vi "Change Sensitivity.vi"(0 "Model in":refnum<class "Model.lvclass">, 5 "Channel":u8, 7 "Offset":sgl, 9 "Sensitivity":sgl, 11 "error in (no error)":errorcluster) -> (4 "Model out":refnum<class "Model.lvclass">, 15 "error out":errorcluster)   [LabVIEW 2016, in "Model.lvclass"]
uses:
  Model.lvclass
  Model.lvclass/Model.ctl
  common_rt_ilc/ILC/ILC.lvclass/ILC.ctl
  common_rt_modbus/DynamicFrameParser/DynamicFrameParser.lvclass
  common_rt_hpilc/HPILC/HPILC.lvclass
  C:/CODE/ts_hpmt/common_rt_ilc/ILC/ILC.lvclass
  Modbus/DesktopModbus/DesktopModbus.lvclass
  common_rt_ilc/ILC/ILC.lvclass
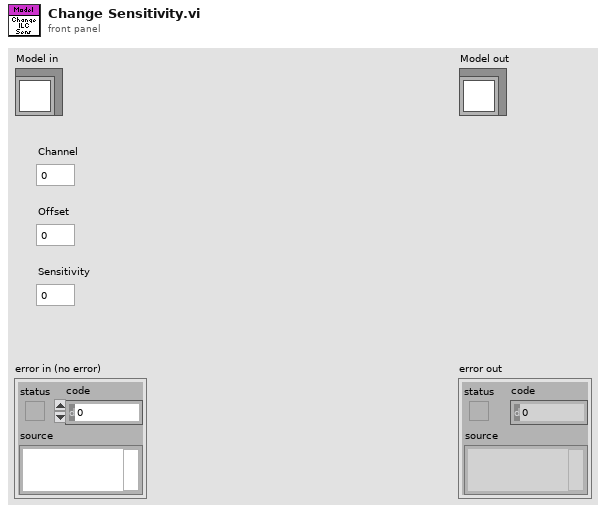
[diagram p1: front panel]
types:
  T1 = typedef "RTILC.lvlib/ILCData.ctl" = cluster{"Constants":T2, "Command":T3, "Telemetry":T5, "Responses":T6, "Timings":T8}
  T2 = typedef "RTILC.lvlib/ILCConstants.ctl" = cluster{"Subnet":u8, "Address":u8}
  T3 = typedef "RTILC.lvlib/ILCCommand.ctl" = cluster{"ILCMode":u16, "TemporaryAddress":u8, "ADCScanRate":T4, "ADCChannel":u8, "ADCOffset":sgl, "ADCSensitivity":sgl}
  T4 = typedef "RTILC.lvlib/ILCScanRates.ctl" = u8
  T5 = typedef "RTILC.lvlib/ILCTelemetry.ctl" = cluster{"UniqueID":u64, "FirmwareType":u8, "NetworkNodeType":u8, "ILCOption":u8, "NetworkNodeOption":u8, "MajorRevision":u8, "MinorRevision":u8, "FirmwareName":string, "ILCMode":u16, "MajorFault":bool, "MinorFault":bool, "FaultOverride":bool, "UniqueIDCRCMismatch":bool, "AppTypeNodeTypeMismatch":bool, "AppMissing":bool, "AppCRCMismatch":bool, "TEDSNotFound":bool, "TEDS1Mismatch":bool, "TEDS2Mismatch":bool, "WatchdogResetDetected":bool, "BrownoutDetected":bool, "EventTrapResetDetected":bool, "TemporaryAddress":u8, "ADCScanRate":T4, "DAC1":u16, "DAC2":u16, "DAC3":u16, "DAC4":u16, "MainADCCalibrationK":sgl[], "MainSensorOffset":sgl[], "MainSensorSensitivity":sgl[], "BackupADCCalibrationK":sgl[], "BackupSensorOffset":sgl[], "BackupSensorSensitivity":sgl[]}
  T6 = typedef "RTILC.lvlib/ILCResponses.ctl" = cluster{"ReportServerID":T7, "ReportServerStatus":T7, "ILCMode":T7, "SetTemporaryAddress":T7, "Reset":T7, "ADCScanRate":T7, "ADCOffsetSensitivity":T7, "ReadDAC":T7, "ReadCalibration":T7}
  T7 = typedef "RTModbus.lvlib/ExceptionCodes.ctl" = u16
  T8 = typedef "RTILC.lvlib/ILCTimings.ctl" = cluster{"ADCOffsetSensitivity":u32, "ADCScanRate":u32, "ILCMode":u32, "ReadCalibration":u32, "ReportServerID":u32, "ReportServerStatus":u32, "Reset":u32, "SetTemporaryAddress":u32}
  T9 = typedef "RTModbus.lvlib/TxFrame.ctl" = cluster{"Data":u8[], "WaitForTrigger":bool, "WaitForRx":u16, "TriggerIRQ":bool, "DelayMicroseconds":u16, "DelayMilliseconds":u16, "Timestamp":bool}
  T10 = typedef "RTModbus.lvlib/RxFrame.ctl" = cluster{"Data":u8[], "Timestamp":u64}
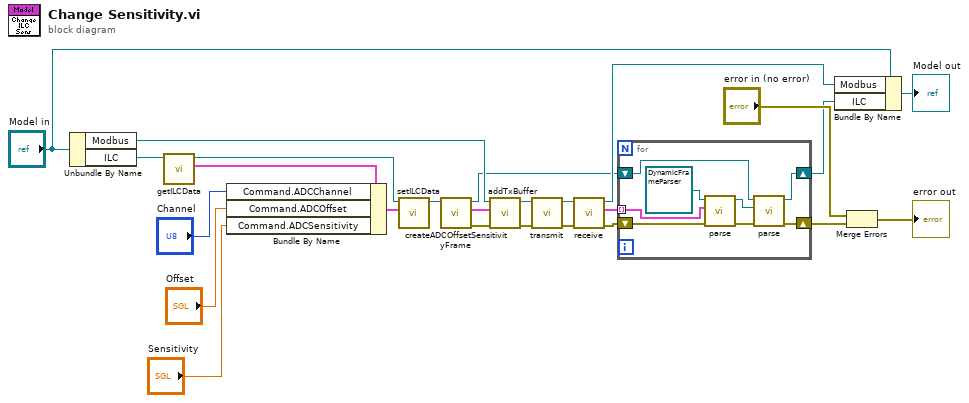
[diagram p0: block diagram]
diagram:
  n1 = Unbundle By Name("Model in") -> ("Modbus"=w19:refnum<class "DesktopModbus.lvclass">, "ILC"=w24:refnum<class "HPILC.lvclass">)
  n2 = call "getILCData.vi"("ILC in"=w24) -> ("ILCData"=w23:T1, "ILC out"=w21:refnum<class "HPILC.lvclass">)  [unwired: 9 in]
  n3 = Bundle By Name(cluster=w23, "Command.ADCChannel"="Channel", "Command.ADCOffset"="Offset", "Command.ADCSensitivity"="Sensitivity") -> (w22:T1)
  n4 = call "setILCData.vi"("ILCData"=w22, "ILC in"=w21) -> ("ILC out"=w20:refnum<class "HPILC.lvclass">)  [unwired: 9 in]
  n5 = call "createADCOffsetSensitivityFrame.vi"("ILC in"=w20) -> ("error out"=w15:errorcluster, "TxFrame"=w18:T9, "ILC out"=w6:refnum<class "HPILC.lvclass">)  [unwired: 8 in]
  n6 = call-dynamic "addTxBuffer.vi"("error in (no error)"=w15, "TxFrame"=w18, "DesktopModbus in"=w19) -> ("error out"=w14:errorcluster, "DesktopModbus out"=w17:refnum<class "DesktopModbus.lvclass">)  [unwired: 7 in]
  n7 = call-dynamic "transmit.vi"("error in (no error)"=w14, "DesktopModbus in"=w17) -> ("error out"=w13:errorcluster, "DesktopModbus out"=w16:refnum<class "DesktopModbus.lvclass">)  [unwired: 8 in]
  n8 = call-dynamic "receive.vi"("error in (no error)"=w13, "DesktopModbus in"=w16) -> ("error out"=w7:errorcluster, "Data"=w8:T10[], "DesktopModbus out"=w10:refnum<class "DesktopModbus.lvclass">)  [unwired: 7 in]
  n9 = for {
    tunnel: w8 -> [w32] mode=indexing
    shift-right: [w26] -> w5
    shift-left: w7 -> [w31]
    shift-right: [w27] -> w4
    shift-left: w6 -> [w28]
    n10 = call "parse.vi"("error in (no error)"=w31, "RxFrame"=w32, "FrameParser in"=refnum<class "DynamicFrameParser.lvclass"> refnum ("RTModbus.lvlib:DynamicFrameParser.lvclass")) -> ("error out"=w30:errorcluster, "FrameParser out"=w29:refnum<class "DynamicFrameParser.lvclass">)  [unwired: 7 in]
    n11 = call-dynamic "parse.vi"("error in (no error)"=w30, "DynamicFrameParser"=w29, "HPILC in"=w28) -> ("error out"=w26:errorcluster, "HPILC out"=w27:refnum<class "HPILC.lvclass">)  [unwired: 6 in, 1 out]
  }
  n12 = Bundle By Name(cluster="Model in", "Modbus"=w10, "ILC"=w4) -> (→"Model out":refnum<class "Model.lvclass">)
  n13 = Merge Errors("error in (no error)", w5) -> (→"error out":errorcluster)
